vi "BIO_write.vi"(8 "error in (no error)":errorcluster, 9 "Timeout (10000ms)":u32=10000, 10 "Bytes to write":u8[](array[numeric]), 11 "BIO in":refnum<class "BIO.lvclass">) -> (0 "error out":errorcluster, 2 "Bytes written":i32, 3 "BIO out":refnum<class "BIO.lvclass">)   [LabVIEW 2013, in "SSL_Lib.lvlib" / "BIO.lvclass"]
uses:
  BIO.lvclass
  SSL-Lib/SSL-Lib.lvclass
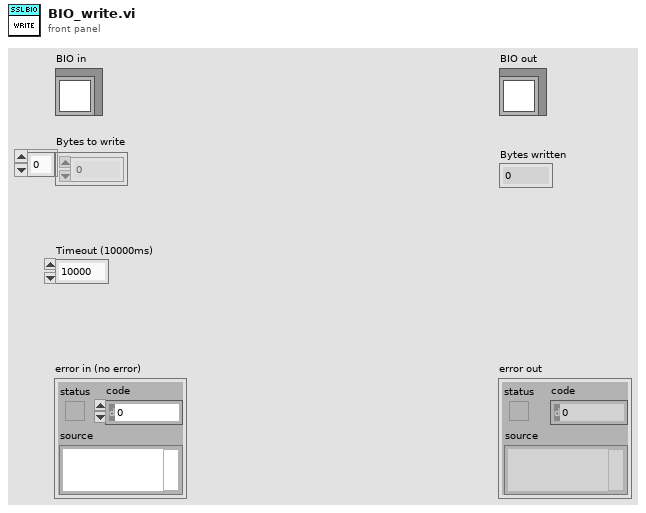
[diagram p1: front panel]
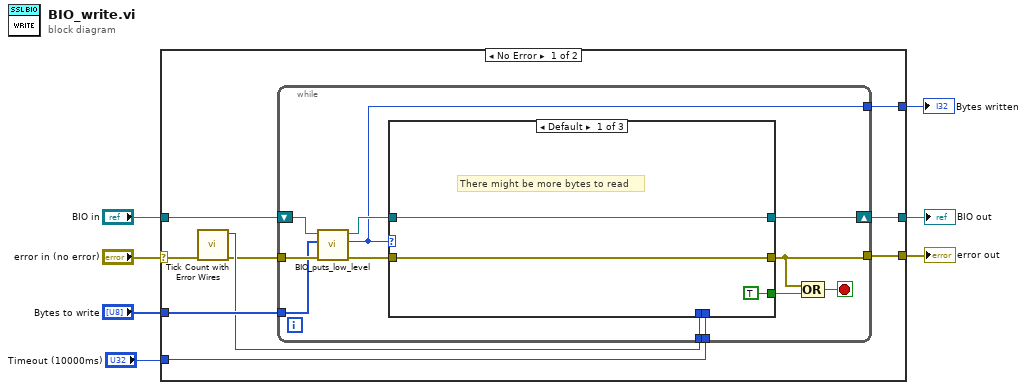
[diagram p0: block diagram]
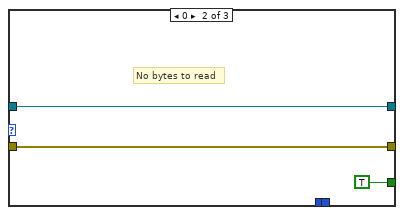
[diagram p2: hidden frame]
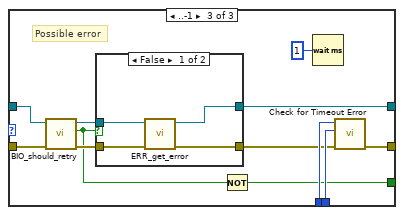
[diagram p3: hidden frame]
diagram:
  n1 = case shown="No Error" "error in (no error)" {
    selector: "error in (no error)" -> [w13 w54]
    tunnel: [w14 w54] -> w6
    tunnel: [w15 w53] -> w4
    tunnel: "BIO in" -> [w9 w53]
    tunnel: "Bytes to write" -> [w16 _]
    tunnel: "Timeout (10000ms)" -> [w11 _]
    tunnel: [w8 _] -> w1
    frame No Error {
      n2 = call "Tick Count with Error Wires.vi"("error in (no error)"=w13) -> ("error out"=w10:errorcluster, "millisecond timer value"=w12:u32)  [unwired: 9 in]
      n3 = while {
        tunnel: w16 -> [w18]
        shift-right: [w26] -> w15
        shift-left: w9 -> [w19]
        tunnel: w10 -> [w28]
        tunnel: [w24] -> w14
        tunnel: w12 -> [w22]
        tunnel: w11 -> [w21]
        tunnel: [w17] -> w8
        stop <- w23 stop-if-true
        n4 = call "BIO_puts_low_level.vi"("error in (no error)"=w28, "Bytes to write"=w18, "BIO in"=w19) -> ("error out"=w27:errorcluster, "return type"=w17:i32, "BIO out"=w20:refnum<class "BIO.lvclass">)  [unwired: 6 in]
        n5 = case shown="Default" w17 {
          tunnel: w27 -> [w30 w34 w46]
          tunnel: [w30 w34 w39] -> w24
          tunnel: w20 -> [w31 w33 w45]
          tunnel: [w31 w33 w42] -> w26
          tunnel: [TRUE ("Should retry") TRUE w35] -> w25
          tunnel: w22 -> [_ _ w40]
          tunnel: w21 -> [_ _ w41]
          frame Default {
            # "There might be more bytes to read"
          }
          frame 0 {
            # "No bytes to read"
          }
          frame ..-1 {
            # "Possible error"
            n6 = call "BIO_should_retry.vi"("error in (no error)"=w46, "BIO in"=w45) -> ("error out"=w44:errorcluster, "Should retry"=w36:bool, "BIO out"=w43:refnum<class "BIO.lvclass">)  [unwired: 7 in]
            n7 = case shown="False" w36 {
              tunnel: w44 -> [w50 w51]
              tunnel: [w49 w51] -> w38
              tunnel: w43 -> [w48 w52]
              tunnel: [w47 w52] -> w42
              frame False {
                n8 = call "ERR_get_error.vi"("error in (no error)"=w50, "SSL-Lib in"=w48) -> ("error out"=w49:errorcluster, "SSL-Lib out"=w47:refnum<class "BIO.lvclass">)  [unwired: 8 in]
              }
              frame True {
              }
            }
            n9 = Not(x=w36) -> (.not. x?=w35:bool)
            n10 = Wait (ms)(milliseconds to wait=u32 1) -> ()  [unwired: 1 out]
            n11 = call "Check for Timeout Error.vi"("error in (no error)"=w38, "Timeout (10000ms)"=w41, "t0"=w40) -> ("error out"=w39:errorcluster)  [unwired: 8 in]
          }
        }
        n12 = Compound Arithmetic op=OR(w24, w25) -> (w23:bool)
      }
    }
    frame Error {
    }
  }
  "error out" <- w6
  "BIO out" <- w4
  "Bytes written" <- w1
